vi "Client.vi"() -> ()   [LabVIEW 2010]
panel:
  in  "Shared Variable Control":refnum<k21>
  in  "stop":bool
  out "String":string
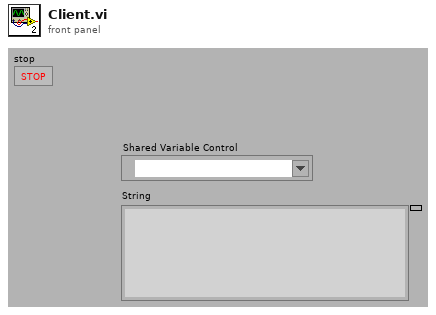
[diagram p1: front panel]
types:
  T1 = enum32{"No PSP", "Read", "Write", "Write & Read"}
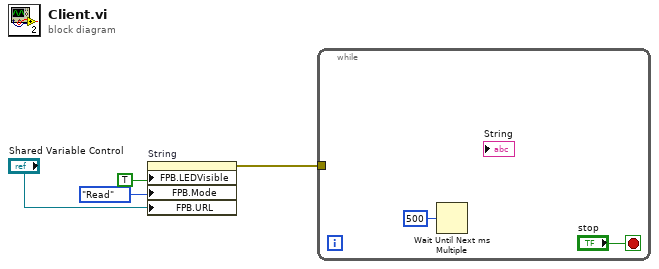
[diagram p0: block diagram]
diagram:
  n1 = property on="String" class="Str"("FPB.LEDVisible"=TRUE ("Data Binding:LED Visible"), "FPB.Mode"=T1."Read" ("Data Binding:Mode"), "FPB.URL"="Shared Variable Control") -> (error out=w2:errorcluster)  [unwired: 2 in, 1 out]
  n2 = while {
    tunnel: w2 -> [_]
    stop <- "stop" stop-if-true
    n3 = Wait Until Next ms Multiple(millisecond multiple=u32 500) -> ()  [unwired: 1 out]
  }
